vi "Delete_Fake_Dots_From_Array([-1,-1...]).vi"(2 "error IN":errorcluster, 3 "Source Array":dbl[][](array[numeric])) -> (0 "error OUT":errorcluster, 1 "Filtered Array (X,Y,dX,dY)":dbl[][](array[numeric]))   [LabVIEW 2013]
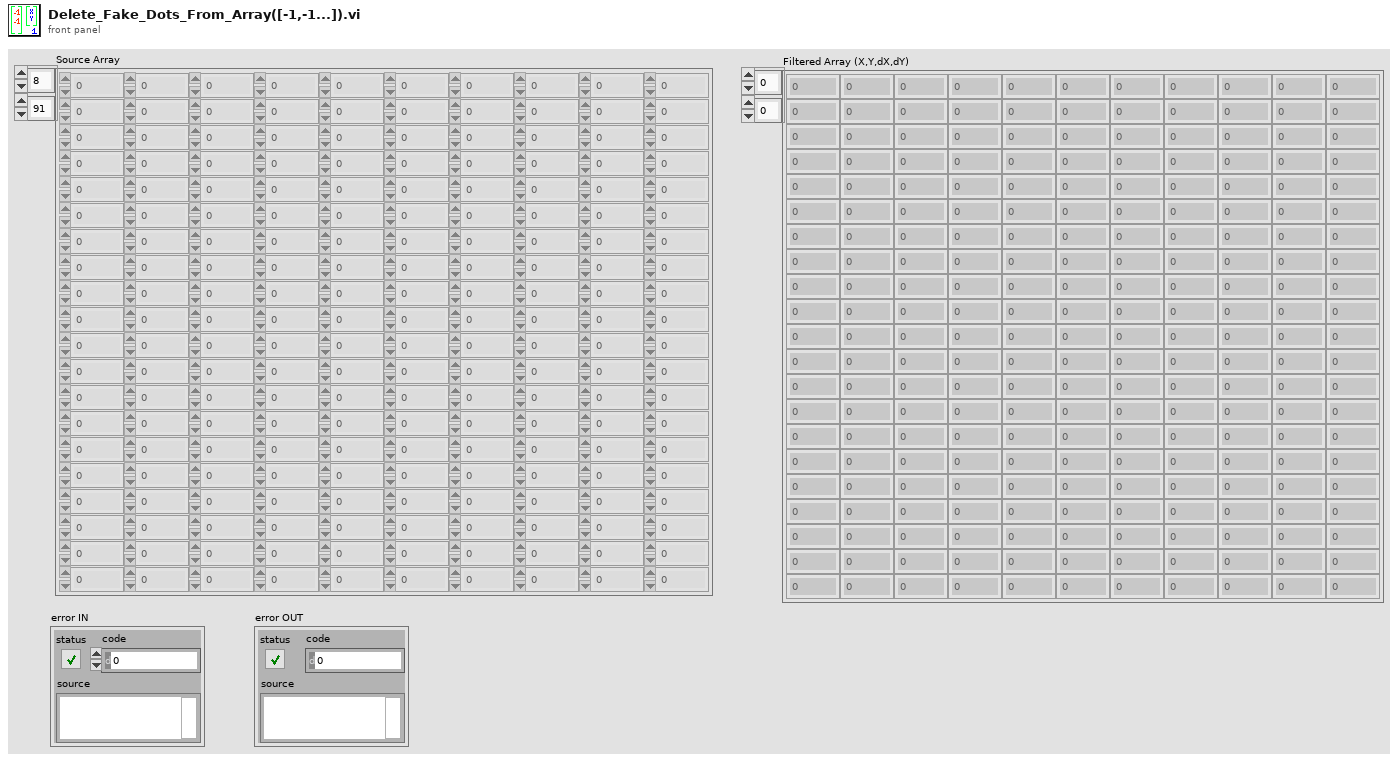
[diagram p1: front panel]
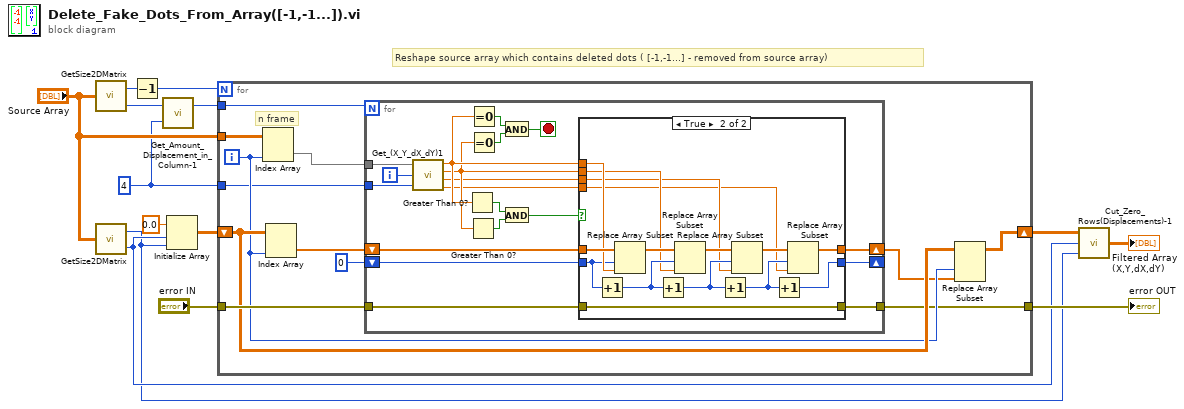
[diagram p0: block diagram]
diagram:
  w1 = 4 ("y")
  # "Reshape source array which contains deleted dots ( [-1,-1...] - removed from source array)"
  n1 = call "GetSize2DMatrix.vi"("Array IN (2D)"="Source Array") -> ("# Cols"=w14:i32, "# Rows"=w3:i32)
  n2 = call "GetSize2DMatrix.vi"("Array IN (2D)"="Source Array") -> ("# Cols"=w5:i32, "# Rows"=w6:i32)
  n3 = Decrement(x=w14) -> (x-1=w13:i32)
  n4 = call "Get_Amount_Displacement_in_Column-1.vi"("multiplier"=w1, "# Rows"=w3) -> ("Displ amount"=w2:i32)  [unwired: 1 out]
  n5 = Initialize Array(0.0 ("element"), w6, w5) -> (w10:dbl[][])
  n6 = for {
    N: w13 -> [_]
    tunnel: "Source Array" -> [w26]
    shift-right: [w21] -> w7
    shift-left: w10 -> [w22]
    tunnel: "error IN" -> [w23]
    tunnel: [w18] -> w8
    tunnel: w2 -> [w16]
    tunnel: w1 -> [w15]
    i -> [w20]
    # "n frame"
    n7 = Index Array(array=w26, index (col)=w20) -> (element=w24:dbl[])  [unwired: 1 in]
    n8 = Index Array(array=w22, index (col)=w20) -> (element=w17:dbl[])  [unwired: 1 in]
    n9 = for {
      N: w16 -> [_]
      tunnel: w24 -> [w45]
      tunnel: w15 -> [w43]
      shift-right: [w29] -> w19
      shift-left: w17 -> [w36]
      shift-right: [w30] -> _
      shift-left: 0 -> [w35]
      tunnel: w23 -> [w28]
      tunnel: [w27] -> w18
      i -> [w44]
      stop <- w40 stop-if-true
      n10 = call "Get_(X_Y_dX_dY)1.vi"("(X,Y,dX,dY)"=w45, "index"=w44, "multiplier"=w43) -> ("X"=w34:dbl, "Y"=w33:dbl, "dX"=w32:dbl, "dY"=w31:dbl)
      n11 = Greater Than 0?(x=w34) -> (x > 0?=w39:bool)
      n12 = Greater Than 0?(x=w33) -> (x > 0?=w38:bool)
      n13 = Equal To 0?(x=w34) -> (x = 0?=w42:bool)
      n14 = Equal To 0?(x=w33) -> (x = 0?=w41:bool)
      n15 = And(x=w42, y=w41) -> (x .and. y?=w40:bool)
      n16 = And(x=w39, y=w38) -> (x .and. y?=w37:bool)
      n17 = case shown="True" w37 {
        tunnel: w36 -> [w48 w63]
        tunnel: w35 -> [w47 w61]
        tunnel: w34 -> [_ w62]
        tunnel: w33 -> [_ w52]
        tunnel: w32 -> [_ w51]
        tunnel: w31 -> [_ w50]
        tunnel: [w47 w54] -> w30
        tunnel: [w48 w53] -> w29
        tunnel: w28 -> [w46 w49]
        tunnel: [w46 w49] -> w27
        frame False {
        }
        frame True {
          n18 = Increment(x=w61) -> (x+1=w59:i32)
          n19 = Replace Array Subset(array=w63, new element=w62, index=w61) -> (w60:dbl[])
          n20 = Increment(x=w59) -> (x+1=w57:i32)
          n21 = Replace Array Subset(array=w60, new element=w52, index=w59) -> (w58:dbl[])
          n22 = Increment(x=w57) -> (x+1=w55:i32)
          n23 = Replace Array Subset(array=w58, new element=w51, index=w57) -> (w56:dbl[])
          n24 = Increment(x=w55) -> (x+1=w54:i32)
          n25 = Replace Array Subset(array=w56, new element=w50, index=w55) -> (w53:dbl[])
        }
      }
    }
    n26 = Replace Array Subset(array=w22, new element=w19, index (col)=w20) -> (w21:dbl[][])  [unwired: 1 in]
  }
  "error OUT" <- w8
  n27 = call "Cut_Zero_Rows(Displacements)-1.vi"("# Cols"=w5, "# Rows"=w6, "Array IN"=w7) -> ("Array OUT"=→"Filtered Array (X,Y,dX,dY)":dbl[][])
